vi "LWXPS_GPIOAnalogGainGet.vi"(8 "LabVIEW error IN":errorcluster, 10 "Analog Input Name":string[](array[string]), 11 "XPS Reference IN":refnum<k24>) -> (0 "XPS Error String":string, 1 "Analog Input Gain Value":i32[](array[numeric]), 2 "Analog Output Name":string[](array[string]), 3 "Returned error code":i32, 4 "LabVIEW error OUT":errorcluster, 5 "XPS Reference OUT":refnum<k24>)   [LabVIEW 2014]
uses:
  D:/XPSQ8_LabView_Library/Development/Source/Dll/Newport.XPS.CommandInterface.dll
  Dll/Newport.XPS.CommandInterface.dll
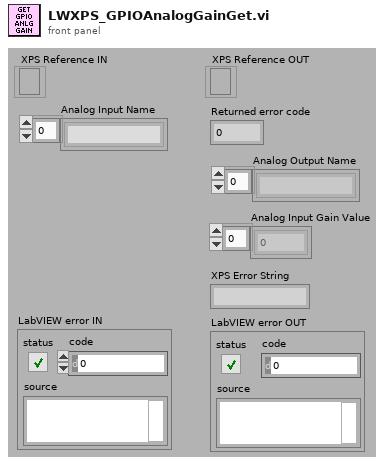
[diagram p1: front panel]
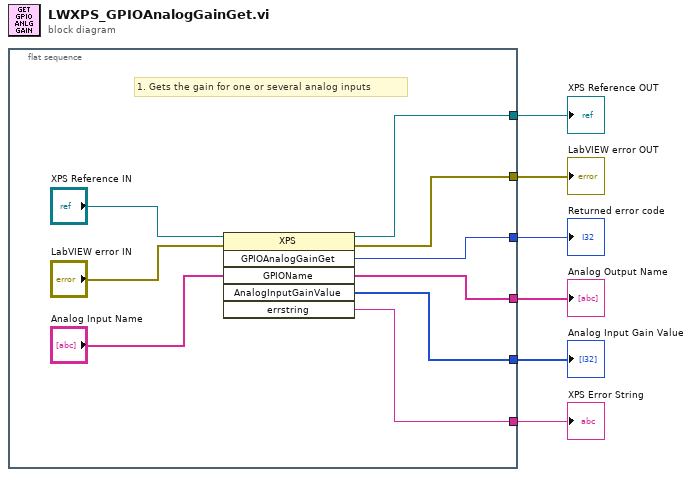
[diagram p0: block diagram]
diagram:
  n1 = flat-sequence {
    tunnel: [w11] -> w6
    tunnel: [w14] -> w5
    tunnel: [w12] -> w4
    tunnel: [w9] -> w1
    tunnel: [w10] -> w2
    tunnel: [w8] -> w3
    frame #0 {
      # "1. Gets the gain for one or several analog inputs"
      n2 = invoke class="XPS" method="GPIOAnalogGainGet"(reference="XPS Reference IN", error in="LabVIEW error IN", "GPIOName"="Analog Input Name") -> (reference out=w11:refnum<k24>, error out=w14:errorcluster, "GPIOAnalogGainGet"=w12:i32, "GPIOName"=w10:string[], "AnalogInputGainValue"=w9:i32[], "errstring"=w8:string)  [unwired: 3 in]
    }
  }
  "XPS Reference OUT" <- w6
  "LabVIEW error OUT" <- w5
  "Returned error code" <- w4
  "XPS Error String" <- w3
  "Analog Output Name" <- w2
  "Analog Input Gain Value" <- w1
